vi "ProcessSensorData.vi"(8 "error in (no error)":errorcluster, 11 "PmuAnalysis":refnum<class "FreqAnalysis.lvclass">) -> (0 "error out":errorcluster, 2 "TimedOut":bool, 3 "PMUAnalysis":refnum<class "FreqAnalysis.lvclass">)   [LabVIEW 2018, in "AnalysisPlugins.lvlib" / "FreqAnalysis.lvclass"]
uses:
  FreqAnalysis.lvclass
  C:/projects/ICDAS/NistPluggableModules/Analysis/AnalysisPlugins/AnalysisPluginBaseClass/AnalysisPluginsBase.lvclass
  C:/projects/ICDAS/NistPluggableModules/Analysis/AnalysisPlugins/PmuAnalysisClass/PmuAnalysis.lvclass
  AnalysisPluginBaseClass/AnalysisPluginsBase.lvclass/AnalysisPluginsBase.ctl
  PmuAnalysisClass/Typedefs/PmuData.ctl
  PmuAnalysisClass/PmuAnalysis.lvclass/PmuAnalysis.ctl
  AnalysisPluginBaseClass/Accessors/Write AnalysisTime.vi
  PmuAnalysisClass/Accessors/Write PmuReport.vi
  AnalysisPluginBaseClass/Accessors/Read SensorQue.vi
  <vilib>/Utility/error.llb/Error Cluster From Error Code.vi
  <vilib>/ErrorRing/Error Ring.xnode
  PmuAnalysisClass/PmuAnalysis.lvclass
panel:
  out "PMU Time Stamp":timestamp format="%^<%.3X\n%x>T"
  out "Waveform Chart":dbl(graph)
  out "Pkt Arrival Time":timestamp format="%^<%.3X\n%x>T"
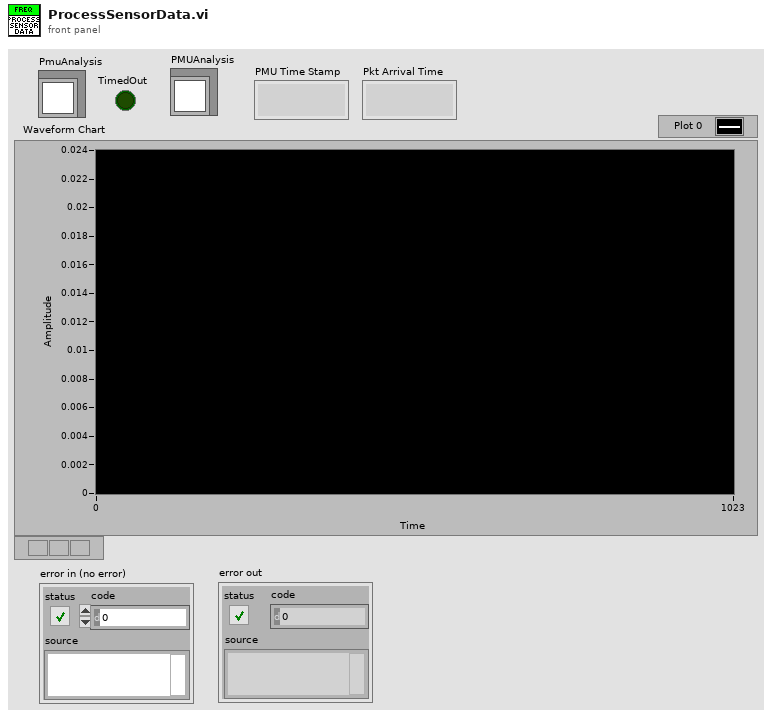
[diagram p1: front panel]
types:
  T1 = typedef "AnalysisPlugins.lvlib/PmuAnalysis.lvclass/PmuData.ctl" = cluster{"Timestamp":dbl, "Synx":cdb[], "Freq":dbl, "ROCOF":dbl, "ID":i16}
  T2 = typedef "SensorQueue.ctl" = refnum<queue>
  T3 = typedef "AnalysisPlugins.lvlib/AnalysisPluginsBase.lvclass/clSensorData.ctl" = cluster{"SensorType":string, "SensorData":variant, "TimeStamp":timestamp}
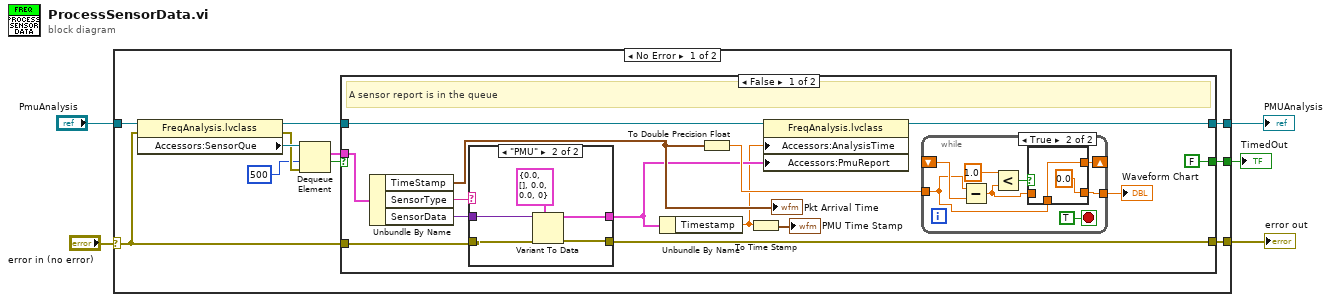
[diagram p0: block diagram]
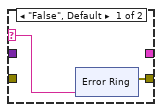
[diagram p3: hidden frame]
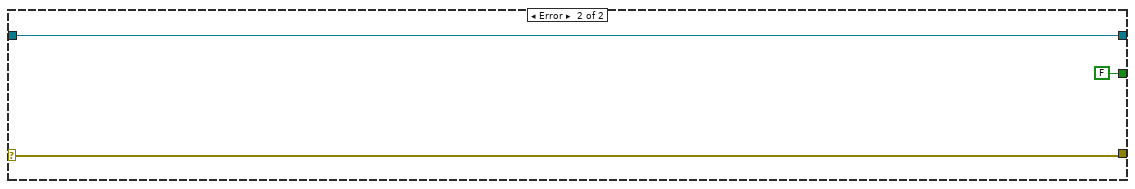
[diagram p5: hidden frame]
diagram:
  n1 = case shown="No Error" "error in (no error)" {
    selector: "error in (no error)" -> [w8 w61]
    tunnel: "PmuAnalysis" -> [w16 w62]
    tunnel: [w15 w62] -> w3
    tunnel: [w14 w61] -> w2
    tunnel: [w6 FALSE] -> w1
    frame No Error {
      n2 = property class="FreqAnalysis.lvclass"(reference=w16, error in=w8) -> (reference out=w13:refnum<class "FreqAnalysis.lvclass">, error out=w11:errorcluster, "Accessors:SensorQue"=w12:T2)
      n3 = Dequeue Element(queue=w12, timeout in ms (-1)=500, error in (no error)=w11) -> (element=w9:T3, timed out?=w7:bool)  [unwired: 2 out]
      n4 = case shown="False" w7 {
        selector: w7 -> [_ w57]
        tunnel: [w28 w59] -> w15
        tunnel: [w27 w58] -> w14
        tunnel: w13 -> [w26 w59]
        tunnel: w9 -> [w25 _]
        tunnel: w8 -> [w23 w58]
        tunnel: [FALSE w57] -> w6
        frame False {
          # "A sensor report is in the queue"
          n5 = Unbundle By Name(w25) -> ("TimeStamp"=w21:timestamp, "SensorType"=w30:string, "SensorData"=w29:variant)
          "Pkt Arrival Time" <- w21
          n6 = case shown="\"PMU\"" w30 {
            selector: w30 -> [w43 _]
            tunnel: [w44 w53] -> w27
            tunnel: w29 -> [_ w56]
            tunnel: w23 -> [_ w55]
            tunnel: [_ w52] -> w19
            frame "False", Default {
              n7 = xnode "Error Ring"("parameter 0"=w43) -> ("error out"=w44:errorcluster)
            }
            frame "PMU" {
              n8 = Variant To Data(error in=w55, type=T1 {"Timestamp"=0.0, "Synx"=[], "Freq"=0.0, "ROCOF"=0.0, "ID"=0} ("PmuReport"), Variant=w56) -> (data=w52:T1, error out=w53:errorcluster)
            }
          }
          n9 = Unbundle By Name(w19) -> ("Timestamp"=w17:dbl)
          n10 = To Double Precision Float(number=w21) -> (double precision float=w20:dbl)
          n11 = To Time Stamp(1:w17) -> (0:→"PMU Time Stamp":timestamp)
          n12 = property class="FreqAnalysis.lvclass"(reference=w26, "Accessors:AnalysisTime"=w17, "Accessors:PmuReport"=w19) -> (reference out=w28:refnum<class "FreqAnalysis.lvclass">)  [unwired: 1 in, 1 out]
          n13 = while {
            tunnel: w20 -> [w32]
            shift-right: [w31] -> _
            shift-left: _ -> [w34]
            tunnel: [w33] -> w24
            stop <- TRUE stop-if-true
            n14 = Subtract(x=w32, y=w34) -> (x-y=w35:dbl)
            n15 = Less?(x=1.0, y=w35) -> (x < y?=w36:bool)
            n16 = case shown="True" w36 {
              tunnel: w35 -> [w40 _]
              tunnel: [w40 0.0] -> w33
              tunnel: w32 -> [w39 w41]
              tunnel: [w39 w41] -> w31
              frame False {
              }
              frame True {
              }
            }
          }
          "Waveform Chart" <- w24
        }
        frame True {
          # "Queue Timed out, allow the loop to run to check for stop state"
        }
      }
    }
    frame Error {
    }
  }
  "PMUAnalysis" <- w3
  "error out" <- w2
  "TimedOut" <- w1
